vi "createNewViFromTemplate.vi"   [LabVIEW 2017, in "create_vi.lvlib"]
doc: "Creates new VI from BenjaminR's VI Template."
uses:
  create_vi.lvlib
  shared/shared.lvlib
types:
  T1 = enum32{"invalid VI type", "Standard VI", "Control VI", "Global VI", "Polymorphic VI", "Configuration VI", "SubSystem", "Facade VI", "Method VI", "Statechart Diagram VI"}
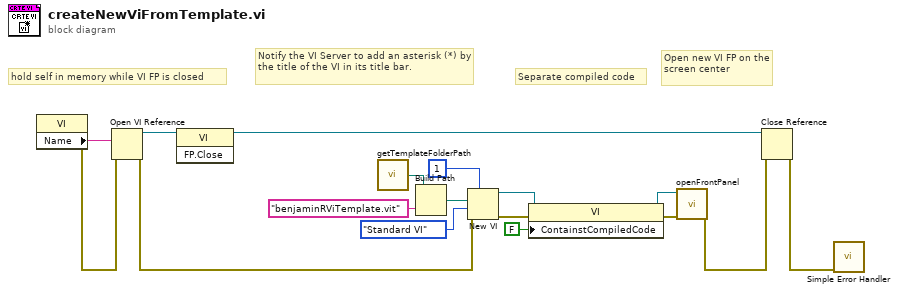
[diagram p0: block diagram]
diagram:
  # "Open new VI FP on the screen center"
  # "Separate compiled code"
  # "Notify the VI Server to add an asterisk (*) by the title of the VI in its title bar."
  # "hold self in memory while VI FP is closed"
  n1 = property class="VI"() -> (error out=w16:errorcluster, "Name"=w17:string)  [unwired: 2 in, 1 out]
  n2 = Open VI Reference(vi path=w17, error in (no error)=w16) -> (vi reference=w3:refnum<vi>, error out=w1:errorcluster)  [unwired: 4 in]
  n3 = invoke class="VI" method="FP.Close"(reference=w3) -> (reference out=w2:refnum<vi>)  [unwired: 2 in, 2 out]
  n4 = call "getTemplateFolderPath.vi"() -> ("Template Folder Path"=w8:path)
  n5 = Build Path(base path=w8, name or relative path="benjaminRViTemplate.vit") -> (appended path=w7:path)
  n6 = New VI(7:u32 1 ("options"), 8:w1, 9:T1."Standard VI" ("vi type (standard vi)"), 10:w7) -> (0:w14:errorcluster, 3:w13:refnum<vi>)  [unwired: 3 in]
  n7 = property class="VI"(reference=w13, error in=w14, "ContainstCompiledCode"=FALSE ("Contains Compiled Code")) -> (reference out=w9:refnum<vi>, error out=w10:errorcluster)
  n8 = call "openFrontPanel.vi"("error in (no error)"=w10, "VI Reference In (Top Level)"=w9) -> ("error out"=w5:errorcluster)  [unwired: 8 in, 1 out]
  n9 = Close Reference(reference=w2, error in (no error)=w5) -> (error out=w4:errorcluster)
  n10 = call <vilib>:"Simple Error Handler.vi"("error in (no error)"=w4) -> ()  [unwired: 4 in, 5 out]
